vi "remove-duplicates.vi"(9 "Input Array":string[](array[string])) -> (1 "Output Array":string[](array[string]), 2 "indices of removed elements":i32[](array[numeric]), 3 "indices of kept elements":i32[](array[numeric]))   [LabVIEW 2014]
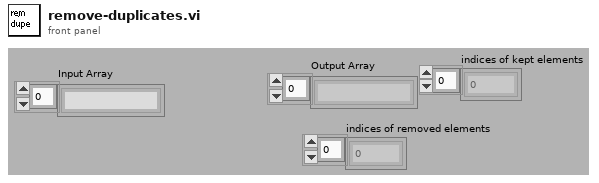
[diagram p1: front panel]
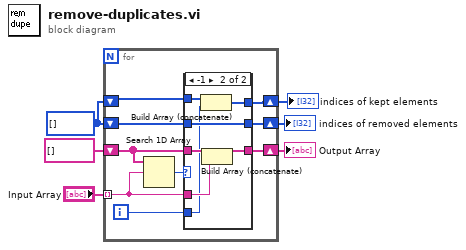
[diagram p0: block diagram]
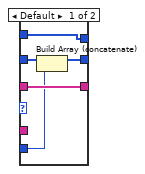
[diagram p2: hidden frame]
diagram:
  w2 = i32[] []
  n1 = for {
    tunnel: "Input Array" -> [w14] mode=indexing
    shift-right: [w13] -> w4
    shift-left: string[] [] -> [w12]
    shift-right: [w10] -> w3
    shift-left: w2 -> [w9]
    shift-right: [w7] -> w1
    shift-left: w2 -> [w8]
    i -> [w11]
    n2 = Search 1D Array(1D array=w12, element=w14) -> (index of element=w15:i32)  [unwired: 1 out]
    n3 = case shown="-1" w15 {
      tunnel: w14 -> [_ w27]
      tunnel: [w20 w25] -> w13
      tunnel: w12 -> [w20 w26]
      tunnel: w11 -> [w17 w23]
      tunnel: [w18 w24] -> w10
      tunnel: w9 -> [w19 w24]
      tunnel: w8 -> [w16 w22]
      tunnel: [w16 w21] -> w7
      frame Default {
        n4 = Build Array (concatenate)(w19, w17) -> (w18:i32[])
      }
      frame -1 {
        n5 = Build Array (concatenate)(w22, w23) -> (w21:i32[])
        n6 = Build Array (concatenate)(w26, w27) -> (w25:string[])
      }
    }
  }
  "Output Array" <- w4
  "indices of removed elements" <- w3
  "indices of kept elements" <- w1
